vi "Operate.vi"(8 "Error_In":errorcluster, 11 "Addition_In":refnum<class "Addition.lvclass">) -> (0 "Error_Out":errorcluster, 3 "Addition_Out":refnum<class "Addition.lvclass">)   [LabVIEW 2023, in "Addition.lvclass"]
doc: "Used to do addition operation by over riding"
uses:
  Addition.lvclass
  D:/Git/Assignments/Assignment-25/Assignment-25_LV_23V/Classes/Calculator/Calculator.lvclass
  Addition.lvclass/Addition.ctl
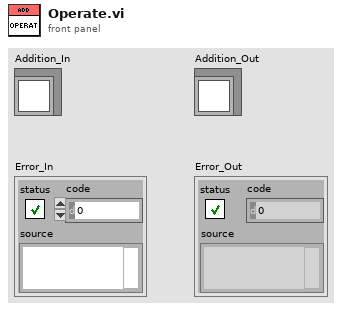
[diagram p1: front panel]
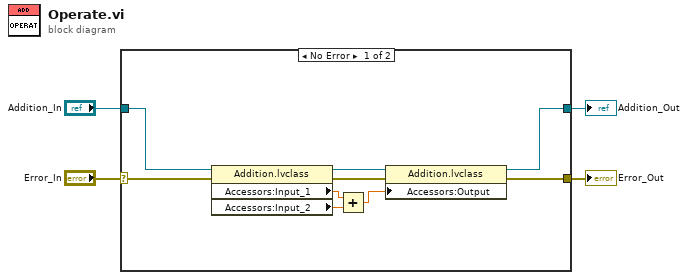
[diagram p0: block diagram]
diagram:
  n1 = case shown="No Error" "Error_In" {
    selector: "Error_In" -> [w13 w15]
    tunnel: [w11 w15] -> w3
    tunnel: [w9 w14] -> w1
    tunnel: "Addition_In" -> [w8 w14]
    frame No Error {
      n2 = property on="Property Node" class="Addition.lvclass"(reference=w8, error in=w13) -> (reference out=w10:refnum<class "Addition.lvclass">, error out=w12:errorcluster, "Accessors:Input_1"=w7:dbl, "Accessors:Input_2"=w6:dbl)
      n3 = Add(x=w7, y=w6) -> (x+y=w5:dbl)
      n4 = property on="Property Node" class="Addition.lvclass"(reference=w10, error in=w12, "Accessors:Output"=w5) -> (reference out=w9:refnum<class "Addition.lvclass">, error out=w11:errorcluster)
    }
    frame Error {
    }
  }
  "Error_Out" <- w3
  "Addition_Out" <- w1
